vi "PC_ParallelThread.vi"(8 "error in (no error)":errorcluster, 11 "VIParameter":T2={"Machine"="192.168.120.8", "VIPath"=path "C:/ni-rt/startup/Test.vi", "Reentrant?"=FALSE, "InputControlName"="InputControl", "InputControlValue"=variant, "OutputControlName"=""}) -> (0 "error out":errorcluster, 3 "VIOutputParameter":T1={"Machine"="192.168.120.8", "VIPath"=path "C:/ni-rt/startup/Test.vi", "Reentrant?"=FALSE, "InputControlName"="InputControl", "InputControlValue"=variant, "OutputControlName"="", "OutputControlValue"=variant})   [LabVIEW 2010]
uses:
  Ctls/PC_DynCallVIParameter.ctl
  Ctls/PC_DynCallVIOutputParameter.ctl
  PC_CallRTGuidedMunitions.vi
  <vilib>/Pansino Software/LabVIEW Architecture/PSARC_Queue Management.llb/PSARC_Queue Insert Element.vi
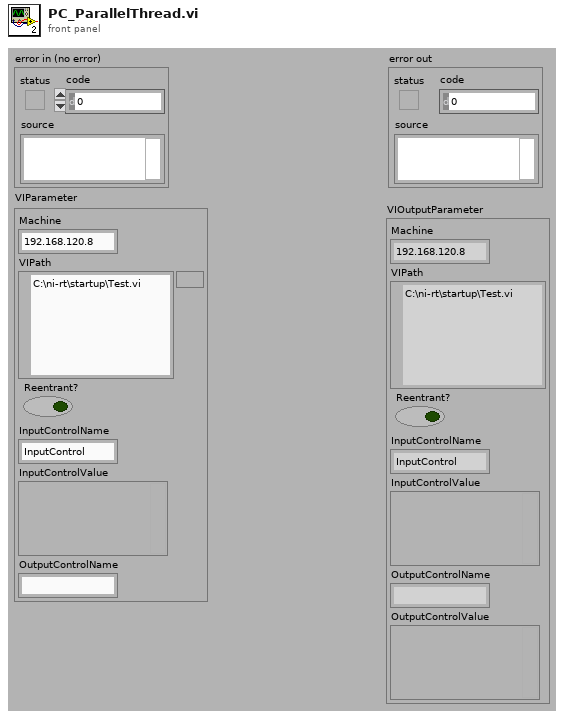
[diagram p1: front panel]
types:
  T1 = typedef "PC_DynCallVIOutputParameter.ctl" = cluster{"Machine":string, "VIPath":path, "Reentrant?":bool, "InputControlName":string, "InputControlValue":variant, "OutputControlName":string, "OutputControlValue":variant}
  T2 = typedef "PC_DynCallVIParameter.ctl" = cluster{"Machine":string, "VIPath":path, "Reentrant?":bool, "InputControlName":string, "InputControlValue":variant, "OutputControlName":string}
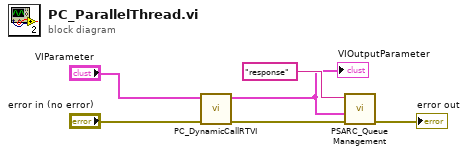
[diagram p0: block diagram]
diagram:
  n1 = call-poly "PC_DynamicCallRTVI.vi"("error in (no error)"="error in (no error)", "VIParameter"="VIParameter") -> ("error out"=w3:errorcluster, "VIOutputParameter"=w1:T1)  [unwired: 8 in]
  "VIOutputParameter" <- w1
  n2 = call-poly <vilib>:"PSARC_Queue Management.vi"("error in (no error)"=w3, "Data"=w1, "Queue Name(unamed)"="response" ("Queue Name")) -> ("error out"=→"error out":errorcluster)  [unwired: 7 in, 1 out]
